vi "Get Job Attribute String.vi"(10 "element":string, 11 "JOB Attributes":string[][](array[string])) -> (3 "Cell String":string)   [LabVIEW 2021]
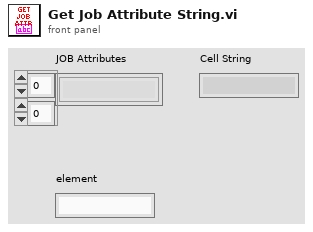
[diagram p1: front panel]
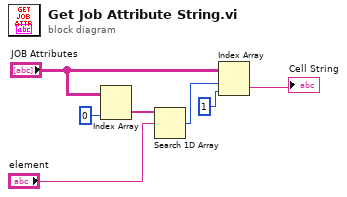
[diagram p0: block diagram]
diagram:
  n1 = Index Array(array="JOB Attributes", index (col)=0 ("disabled index (col)")) -> (element=w2:string[])  [unwired: 1 in]
  n2 = Search 1D Array(1D array=w2, element="element") -> (index of element=w5:i32)  [unwired: 1 in]
  n3 = Index Array(array="JOB Attributes", index (row)=w5, index (col)=1 ("disabled index (col)")) -> (element=→"Cell String":string)
